vi "ke37xx Configure Measurement.vi"(0 "VISA Resource Name":refnum<visa-resource-name>, 5 "Function (0: None)":T2(ring), 7 "Auto Range (T: On)":bool=TRUE, 9 "Auto Zero (1: On)":enum16{"Off", "On", "Once"}(ring)=enum."On", 11 "error in (no error)":errorcluster, 12 "Manual Range":dbl, 13 "DMM Connection (1: All)":T1(ring)=enum."All") -> (4 "VISA Resource Name Out":refnum<visa-resource-name>, 15 "error out":errorcluster)   [LabVIEW 2009, in "Keithley 3700 Series.lvlib"]
doc: "This VI allows you to configure various aspects of the measurement system."
uses:
  <instrlib>/Keithley 3706/Keithley 3700 Series.lvlib
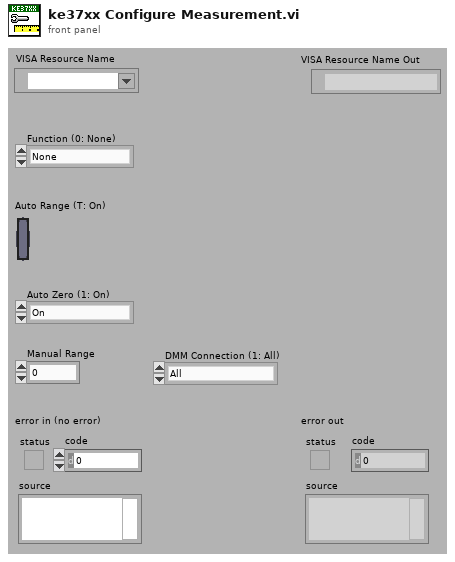
[diagram p1: front panel]
types:
  T1 = enum16{"None", "All", "2-Wire", "4-Wire", "2-Wire Amps", "Amps"}
  T2 = enum16{"None", "DC Volts", "AC Volts", "DC Current", "AC Current", "2-Wire Ohms", "4-Wire Ohms", "Temperature", "Period", "Frequency", "Continuity", "Commonside Ohms"}
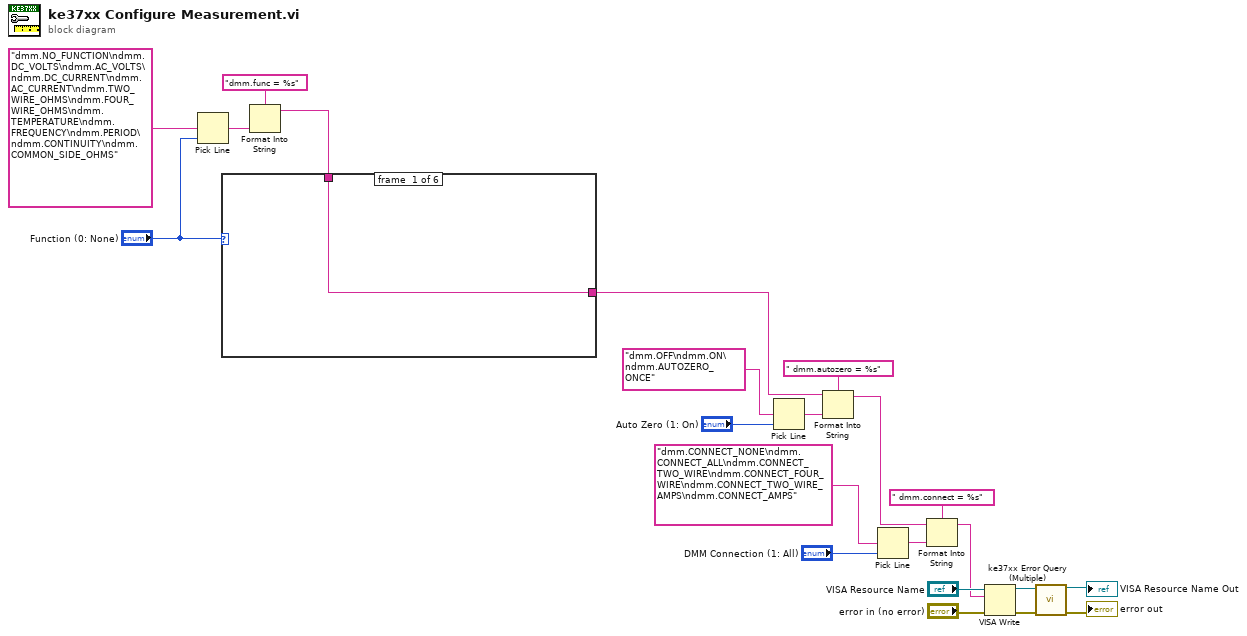
[diagram p0: block diagram]
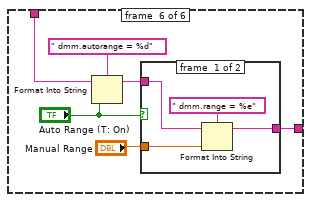
[diagram p6: hidden frame]
diagram:
  n1 = Pick Line(multi-line string="dmm.NO_FUNCTION\ndmm.DC_VOLTS\ndmm.AC_VOLTS\ndmm.DC_CURRENT\ndmm.AC_CURRENT\ndmm.TWO_WIRE_OHMS\ndmm.FOUR_WIRE_OHMS\ndmm.TEMPERATURE\ndmm.FREQUENCY\ndmm.PERIOD\ndmm.CONTINUITY\ndmm.COMMON_SIDE_OHMS", line index="Function (0: None)") -> (output string=w12:string)  [unwired: 1 out]
  n2 = Format Into String(format string="dmm.func = %s" ("write buffer"), w12) -> (resulting string=w4:string)  [unwired: 2 in, 1 out]
  n3 = case shown="Default" "Function (0: None)" {
    tunnel: w4 -> [w23 w24 w25 w26 w27 w29]
    tunnel: [w23 w24 w25 w26 w27 w28] -> w3
    frame #0 {
    }
    frame #1 {
    }
    frame #2 {
    }
    frame #3 {
    }
    frame #4 {
    }
    frame #5 {
      n4 = Format Into String(format string=" dmm.autorange = %d" ("true string"), initial string=w29, "Auto Range (T: On)") -> (resulting string=w30:string)  [unwired: 1 in, 1 out]
      n5 = case shown="False" "Auto Range (T: On)" {
        tunnel: w30 -> [w36 w38]
        tunnel: "Manual Range" -> [w35 _]
        tunnel: [w34 w38] -> w28
        frame #0 {
          n6 = Format Into String(format string=" dmm.range = %e" ("true string"), initial string=w36, w35) -> (resulting string=w34:string)  [unwired: 1 in, 1 out]
        }
        frame #1 {
        }
      }
    }
  }
  n7 = Pick Line(multi-line string="dmm.OFF\ndmm.ON\ndmm.AUTOZERO_ONCE", line index="Auto Zero (1: On)") -> (output string=w14:string)  [unwired: 1 out]
  n8 = Format Into String(format string=" dmm.autozero = %s" ("write buffer"), initial string=w3, w14) -> (resulting string=w5:string)  [unwired: 1 in, 1 out]
  n9 = Pick Line(multi-line string="dmm.CONNECT_NONE\ndmm.CONNECT_ALL\ndmm.CONNECT_TWO_WIRE\ndmm.CONNECT_FOUR_WIRE\ndmm.CONNECT_TWO_WIRE_AMPS\ndmm.CONNECT_AMPS", line index="DMM Connection (1: All)") -> (output string=w9:string)  [unwired: 1 out]
  n10 = Format Into String(format string=" dmm.connect = %s" ("write buffer"), initial string=w5, w9) -> (resulting string=w2:string)  [unwired: 1 in, 1 out]
  n11 = VISA Write(VISA resource name="VISA Resource Name", write buffer=w2, error in (no error)="error in (no error)") -> (VISA resource name out=w18:refnum<visa-resource-name>, error out=w17:errorcluster)  [unwired: 1 out]
  n12 = call <instrlib>:"ke37xx Error Query (Multiple).vi"("VISA resource name"=w18, "error in (no error)"=w17) -> ("VISA resource name out"=→"VISA Resource Name Out":refnum<visa-resource-name>, "error out"=→"error out":errorcluster)  [unwired: 12 out]
